vi "Get Initial Stock Levels.vi"() -> (2 "Stock":T1[](array[typedef]))   [LabVIEW 2019, in "Stock.lvlib"]
uses:
  Stock.lvlib
  Products.ctl
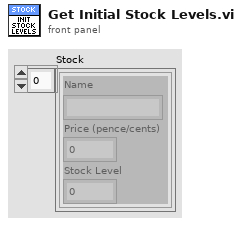
[diagram p1: front panel]
types:
  T1 = typedef "Stock.lvlib/Products.ctl" = cluster{"Name":string, "Price (pence/cents)":u32, "Stock Level":u32}
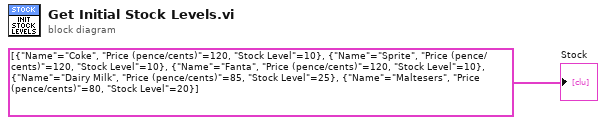
[diagram p0: block diagram]
diagram:
  "Stock" <- T1[] [{"Name"="Coke", "Price (pence/cents)"=120, "Stock Level"=10}, {"Name"="Sprite", "Price (pence/cents)"=120, "Stock Level"=10}, {"Name"="Fanta", "Price (pence/cents)"=120, "Stock Level"=10}, {"Name"="Dairy Milk", "Price (pence/cents)"=85, "Stock Level"=25}, {"Name"="Maltesers", "Price (pence/cents)"=80, "Stock Level"=20}] ("Stock")
